vi "EF_EstimateEntropy.vi"(0 "Array in":dbl[](array[numeric]), 1 "X max":dbl=100.0 format="%0.2f", 2 "X min":dbl=-100.0 format="%0.2f", 3 "# bins":i32=100, 4 "Normalized ?":bool) -> (5 "Shannon Entropy out":dbl)   [LabVIEW 2016, in "Feature Extraction.lvlib"]
uses:
  Feature Extraction.lvlib
  <vilib>/Analysis/NI_AALPro.lvlib
panel:
  # "This VI is a part of BCI Design library, http://www.ru-bci.org \nCopyright © 2020, Sotnikov Peter, All rights reserved. License: GNU GPLv3"
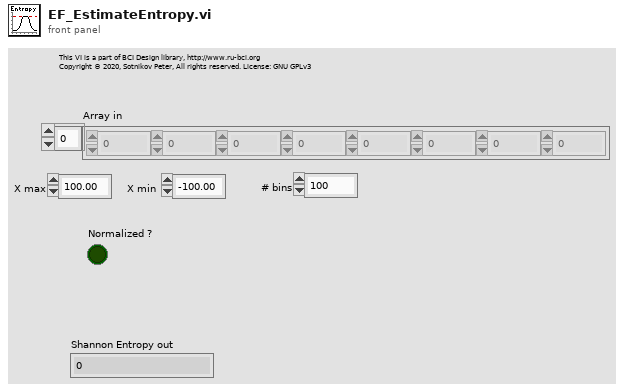
[diagram p1: front panel]
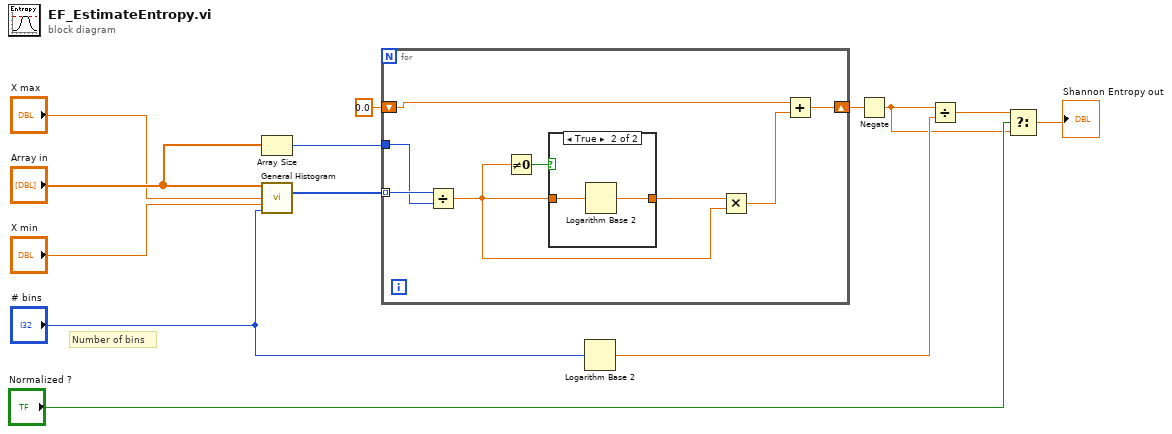
[diagram p0: block diagram]
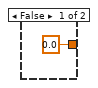
[diagram p2: hidden frame]
diagram:
  # "Number of bins"
  n1 = Array Size(array="Array in") -> (size(s)=w11:i32)
  n2 = call <vilib>:"General Histogram.vi"("X"="Array in", "max"="X max", "min"="X min", "# bins"="# bins") -> ("Histogram"=w12:i32[])  [unwired: 7 in, 4 out]
  n3 = for {
    tunnel: w12 -> [w21] mode=indexing
    tunnel: w11 -> [w20]
    shift-right: [w18] -> w9
    shift-left: 0.0 -> [w17]
    n4 = Divide(x=w21, y=w20) -> (x/y=w14:dbl)
    n5 = Not Equal To 0?(x=w14) -> (x != 0?=w15:bool)
    n6 = case shown="True" w15 {
      tunnel: [0.0 w24] -> w19
      tunnel: w14 -> [_ w23]
      frame False {
      }
      frame True {
        n7 = Logarithm Base 2(1:w23) -> (0:w24:dbl)
      }
    }
    n8 = Multiply(x=w19, y=w14) -> (x*y=w16:dbl)
    n9 = Add(x=w17, y=w16) -> (x+y=w18:dbl)
  }
  n10 = Logarithm Base 2(1:"# bins") -> (0:w5:dbl)
  n11 = Negate(x=w9) -> (-x=w1:dbl)
  n12 = Divide(x=w1, y=w5) -> (x/y=w2:dbl)
  n13 = Select(t=w2, s="Normalized ?", f=w1) -> (s? t:f=→"Shannon Entropy out":dbl)
